vi "shujudaa.vi"(1 "量程-1":T1(ring), 2 "inputdata":i32[](array[numeric])) -> (0 "outdata":dbl[](array[numeric]))   [LabVIEW 2012]
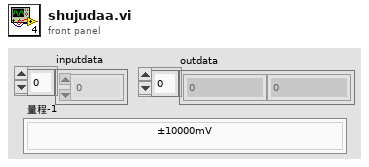
[diagram p1: front panel]
types:
  T1 = enum16{"±10000mV", "±5000mV", "±2500mV", "0-10000mV", "0-5000mV"}
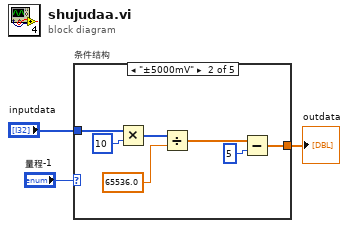
[diagram p0: block diagram]
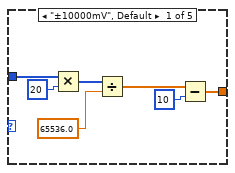
[diagram p2: hidden frame]
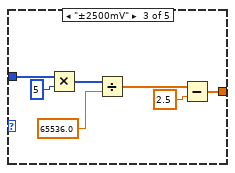
[diagram p3: hidden frame]
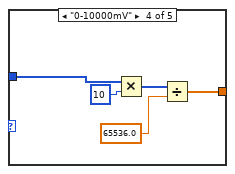
[diagram p4: hidden frame]
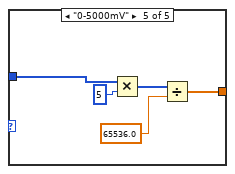
[diagram p5: hidden frame]
diagram:
  n1 = case "条件结构" shown="\"±5000mV\"" "量程-1" {
    tunnel: "inputdata" -> [w10 w12 w19 w26 w31]
    tunnel: [w4 w11 w18 w25 w30] -> w2
    frame "±10000mV", Default {
      n2 = Multiply(x=w10, y=20) -> (x*y=w7:i32[])
      n3 = Divide(x=w7, y=65536.0) -> (x/y=w6:dbl[])
      n4 = Subtract(x=w6, y=10) -> (x-y=w4:dbl[])
    }
    frame "±5000mV" {
      n5 = Multiply(x=w12, y=10) -> (x*y=w15:i32[])
      n6 = Divide(x=w15, y=65536.0) -> (x/y=w14:dbl[])
      n7 = Subtract(x=w14, y=5) -> (x-y=w11:dbl[])
    }
    frame "±2500mV" {
      n8 = Multiply(x=w19, y=5) -> (x*y=w22:i32[])
      n9 = Divide(x=w22, y=65536.0) -> (x/y=w21:dbl[])
      n10 = Subtract(x=w21, y=2.5) -> (x-y=w18:dbl[])
    }
    frame "0-10000mV" {
      n11 = Multiply(x=w26, y=10) -> (x*y=w27:i32[])
      n12 = Divide(x=w27, y=65536.0) -> (x/y=w25:dbl[])
    }
    frame "0-5000mV" {
      n13 = Multiply(x=w31, y=5) -> (x*y=w32:i32[])
      n14 = Divide(x=w32, y=65536.0) -> (x/y=w30:dbl[])
    }
  }
  "outdata" <- w2
